vi "Scripting_SetConnectorPanePattern.vi"(0 "VIPath(s)/ViRef(s)":variant, 1 "Pattern":T1 items=["4x4x4", "5x6x5", "6x8x6"], 2 "UpdateCallersInThisClassOnly":string, 5 "error in (no error)":errorcluster, 6 "AppRef":refnum<vi>) -> (19 "error out":errorcluster)   [LabVIEW 2020]
uses:
  Scripting_ConnectorPanePatternType.ctl
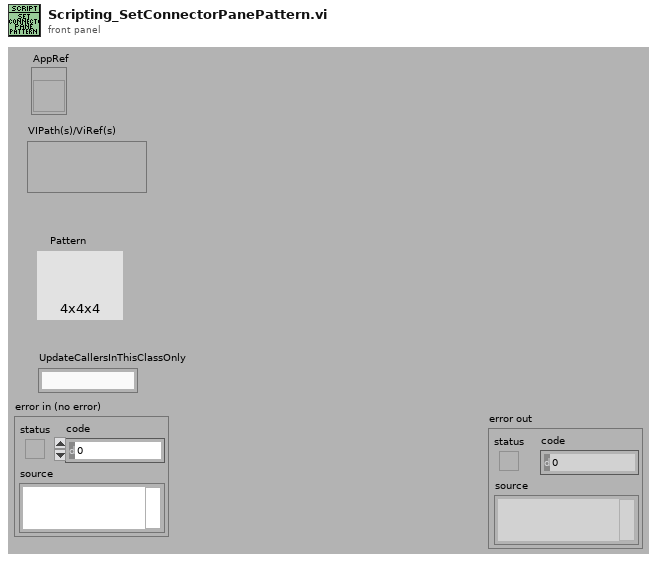
[diagram p1: front panel]
types:
  T1 = typedef "Scripting_ConnectorPanePatternType.ctl" = u16
  T2 = enum32{"invalid lock state", "Not Locked", "Locked (No Password)", "Password-protected"}
  T3 = enum32{"invalid VI type", "Standard VI", "Control VI", "Global VI", "Polymorphic VI", "Configuration VI", "SubSystem", "Facade VI", "Method VI", "Statechart Diagram VI"}
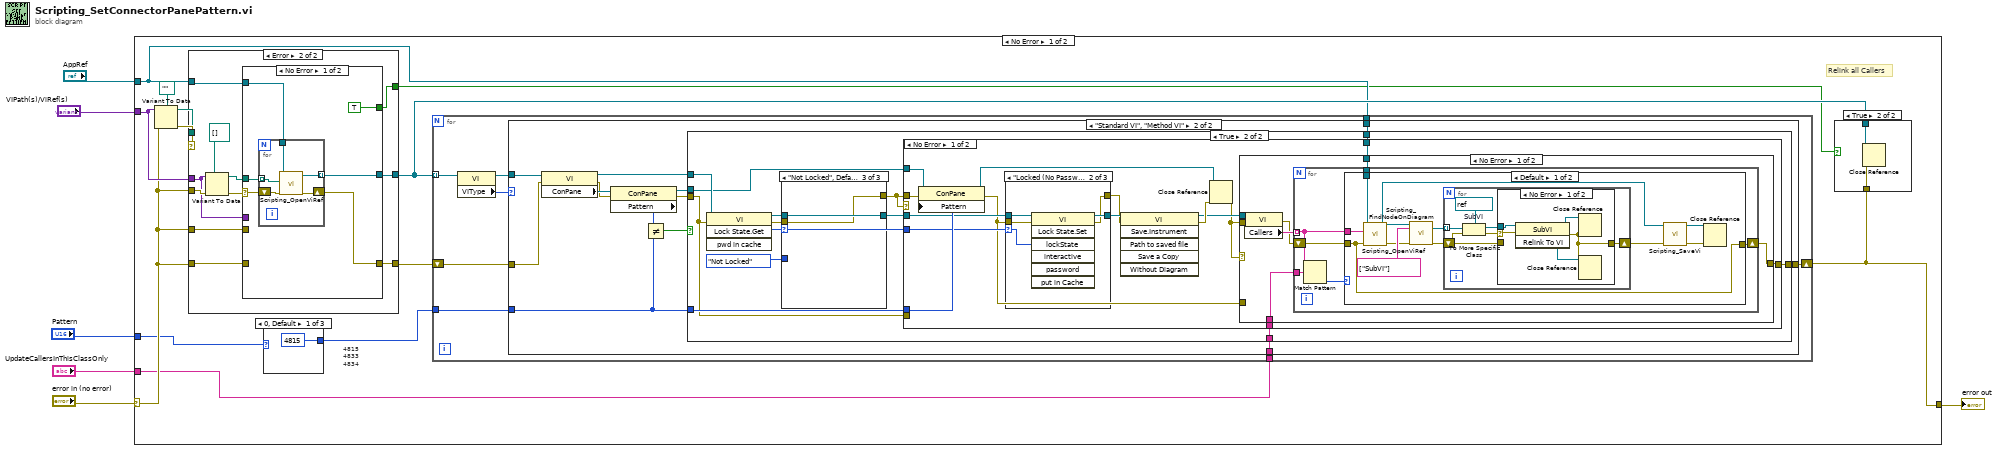
[diagram p0: block diagram]
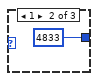
[diagram p3: hidden frame]
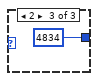
[diagram p4: hidden frame]
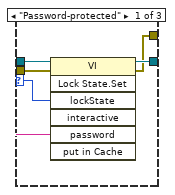
[diagram p10: hidden frame]
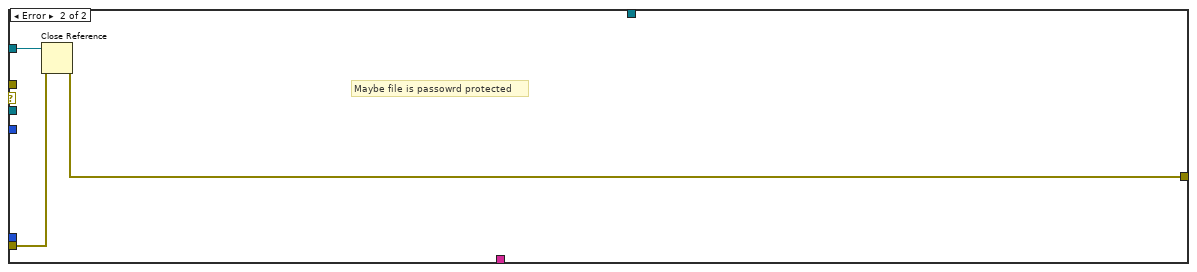
[diagram p12: hidden frame]
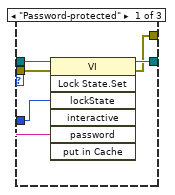
[diagram p13: hidden frame]
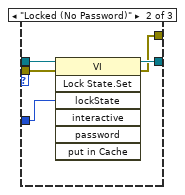
[diagram p14: hidden frame]
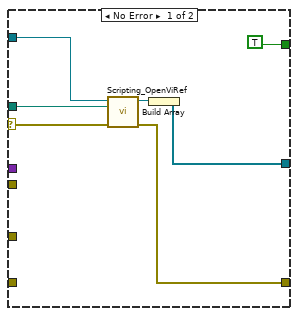
[diagram p15: hidden frame]
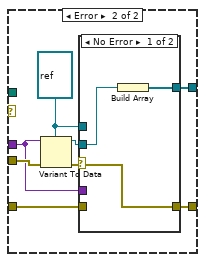
[diagram p16: hidden frame]
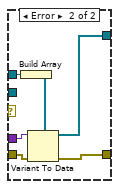
[diagram p17: hidden frame]
diagram:
  n1 = case shown="No Error" "error in (no error)" {
    selector: "error in (no error)" -> [w15 w189]
    tunnel: "VIPath(s)/ViRef(s)" -> [w17 _]
    tunnel: "Pattern" -> [w14 _]
    tunnel: [w8 w189] -> w3
    tunnel: "UpdateCallersInThisClassOnly" -> [w10 _]
    tunnel: "AppRef" -> [w9 _]
    frame No Error {
      # "Relink all Callers"
      # "4815\n4833\n4834"
      n2 = Variant To Data(error in=w15, type=path "", Variant=w17) -> (data=w16:path, error out=w18:errorcluster)
      n3 = case shown="Error" w18 {
        selector: w18 -> [w148 _]
        tunnel: w17 -> [_ w155]
        tunnel: w16 -> [w149 _]
        tunnel: [w146 w157] -> w11
        tunnel: w15 -> [_ w156]
        tunnel: w15 -> [_ w154]
        tunnel: w15 -> [_ w153]
        tunnel: [w145 w152] -> w12
        tunnel: [TRUE w151] -> w7
        tunnel: w9 -> [w143 w150]
        frame No Error {
          n4 = call "Scripting_OpenViRef.vi"("error in"=w148, "ViPath/ViName/Viref"=w149, "AppRef"=w143) -> ("error out"=w145:errorcluster, "vi reference"=w147:refnum<vi>)  [unwired: 6 in, 1 out]
          n5 = Build Array(w147) -> (w146:refnum<vi>[])
        }
        frame Error {
          n6 = Variant To Data(error in=w156, type=path[] [], Variant=w155) -> (data=w158:path[], error out=w159:errorcluster)
          n7 = case shown="No Error" w159 {
            selector: w159 -> [w164 _]
            tunnel: w158 -> [w166 _]
            tunnel: [w165 w177] -> w157
            tunnel: w155 -> [_ w174]
            tunnel: w154 -> [_ w179]
            tunnel: w153 -> [_ w175]
            tunnel: [w163 w172] -> w152
            tunnel: [TRUE _] -> w151
            tunnel: w150 -> [w161 _]
            frame No Error {
              n8 = for {
                tunnel: w166 -> [w171] mode=indexing
                tunnel: [w170] -> w165 mode=indexing
                shift-right: [w168] -> w163
                shift-left: w164 -> [w169]
                tunnel: w161 -> [w167]
                n9 = call "Scripting_OpenViRef.vi"("error in"=w169, "ViPath/ViName/Viref"=w171, "AppRef"=w167) -> ("error out"=w168:errorcluster, "vi reference"=w170:refnum<vi>)  [unwired: 6 in, 1 out]
              }
            }
            frame Error {
              w173 = refnum<vi> refnum ("Reference")
              n10 = Variant To Data(error in=w179, type=w173, Variant=w174) -> (data=w178:refnum<vi>, error out=w176:errorcluster)
              n11 = case shown="No Error" w176 {
                selector: w176 -> [w180 _]
                tunnel: w178 -> [w182 _]
                tunnel: [w181 w184] -> w177
                tunnel: w175 -> [_ w188]
                tunnel: w174 -> [_ w187]
                tunnel: w173 -> [_ w186]
                tunnel: [w180 w183] -> w172
                frame No Error {
                  n12 = Build Array(w182) -> (w181:refnum<vi>[])
                }
                frame Error {
                  n13 = Build Array(w186) -> (w185:refnum<vi>[])
                  n14 = Variant To Data(error in=w188, type=w185, Variant=w187) -> (data=w184:refnum<vi>[], error out=w183:errorcluster)
                }
              }
            }
          }
        }
      }
      n15 = case shown="0, Default" w14 {
        tunnel: [u32 4815 ("Pattern") u32 4833 ("Pattern") u32 4834 ("Pattern")] -> w13
        frame 0, Default {
        }
        frame 1 {
        }
        frame 2 {
        }
      }
      n16 = for {
        tunnel: w11 -> [w29] mode=indexing
        tunnel: w13 -> [w30]
        shift-right: [w31] -> w8
        shift-left: w12 -> [w32]
        tunnel: w10 -> [w26]
        tunnel: w9 -> [w25]
        n17 = property class="VI"(reference=w29) -> (reference out=w28:refnum<vi>, "VIType"=w27:T3)  [unwired: 1 in, 1 out]
        n18 = case shown="\"Standard VI\", \"Method VI\"" w27 {
          tunnel: w32 -> [w33 w42]
          tunnel: [w33 w39] -> w31
          tunnel: w30 -> [_ w38]
          tunnel: w28 -> [_ w37]
          tunnel: w26 -> [_ w35]
          tunnel: w25 -> [_ w34]
          frame "invalid VI type", "Control VI", "Polymorphic VI", Default {
          }
          frame "Standard VI", "Method VI" {
            n19 = property class="VI"(reference=w37, error in=w42) -> (reference out=w36:refnum<vi>, error out=w43:errorcluster, "ConPane"=w46:refnum<vi>)
            n20 = property class="ConPane"(reference=w46, error in=w43) -> (reference out=w45:refnum<vi>, error out=w44:errorcluster, "Pattern"=w41:u32)
            n21 = Not Equal?(x=w41, y=w38) -> (x != y?=w40:bool)
            n22 = case shown="True" w40 {
              tunnel: w45 -> [_ w55]
              tunnel: w44 -> [w47 w50]
              tunnel: [w47 w52] -> w39
              tunnel: w38 -> [_ w60]
              tunnel: w36 -> [_ w59]
              tunnel: w35 -> [_ w49]
              tunnel: w34 -> [_ w48]
              frame False {
              }
              frame True {
                n23 = invoke class="VI" method="Lock State.Get"(reference=w59, error in=w50) -> (reference out=w58:refnum<vi>, error out=w57:errorcluster, "Get Lock State"=w54:T2)  [unwired: 2 in, 1 out]
                n24 = case shown="\"Not Locked\", Default" w54 {
                  tunnel: w58 -> [w135 w140 w142]
                  tunnel: w57 -> [w134 w139 w141]
                  tunnel: T2."Not Locked" ("Lock State") -> [w133 w138 _]
                  tunnel: [w131 w137 w142] -> w53
                  tunnel: [w130 w136 w141] -> w51
                  frame "Password-protected" {
                    n25 = invoke class="VI" method="Lock State.Set"(reference=w135, error in=w134, "lockState"=w133, "password"="Endevo Knows Goop!" ("Password")) -> (reference out=w131:refnum<vi>, error out=w130:errorcluster)  [unwired: 3 in, 5 out]
                  }
                  frame "Locked (No Password)" {
                    (unwired) "Endevo Knows Goop!" ("Password")
                    n26 = invoke class="VI" method="Lock State.Set"(reference=w140, error in=w139, "lockState"=w138) -> (reference out=w137:refnum<vi>, error out=w136:errorcluster)  [unwired: 4 in, 5 out]
                  }
                  frame "Not Locked", Default {
                  }
                }
                n27 = case shown="No Error" w51 {
                  tunnel: w60 -> [w75 _]
                  tunnel: w51 -> [w74 _]
                  tunnel: w55 -> [w73 w129]
                  tunnel: w54 -> [w72 _]
                  tunnel: w53 -> [w67 _]
                  tunnel: [w65 w127] -> w52
                  tunnel: w50 -> [_ w128]
                  tunnel: w49 -> [w62 _]
                  tunnel: w48 -> [w61 _]
                  frame No Error {
                    n28 = property class="ConPane"(reference=w73, error in=w74, "Pattern"=w75) -> (reference out=w68:refnum<vi>, error out=w63:errorcluster)
                    n29 = case shown="\"Locked (No Password)\"" w72 {
                      selector: w72 -> [w114 w120 _]
                      tunnel: w67 -> [w119 w124 w126]
                      tunnel: w63 -> [w118 w123 w125]
                      tunnel: [w116 w122 w126] -> w71
                      tunnel: [w115 w121 w125] -> w70
                      frame "Password-protected" {
                        n30 = invoke class="VI" method="Lock State.Set"(reference=w119, error in=w118, "lockState"=w114, "password"="Endevo Knows Goop!" ("Password")) -> (reference out=w116:refnum<vi>, error out=w115:errorcluster)  [unwired: 3 in, 5 out]
                      }
                      frame "Locked (No Password)" {
                        (unwired) "Endevo Knows Goop!" ("Password")
                        n31 = invoke class="VI" method="Lock State.Set"(reference=w124, error in=w123, "lockState"=w120) -> (reference out=w122:refnum<vi>, error out=w121:errorcluster)  [unwired: 4 in, 5 out]
                      }
                      frame "Not Locked", Default {
                      }
                    }
                    n32 = invoke class="VI" method="Save.Instrument"(reference=w71, error in=w70) -> (reference out=w66:refnum<vi>, error out=w69:errorcluster)  [unwired: 4 in, 4 out]
                    n33 = Close Reference(reference=w68, error in (no error)=w69) -> (error out=w64:errorcluster)
                    n34 = case shown="No Error" w64 {
                      tunnel: w66 -> [w82 _]
                      tunnel: w64 -> [w81 _]
                      tunnel: [w78 w113] -> w65
                      tunnel: w63 -> [_ w113]
                      tunnel: w62 -> [w77 _]
                      tunnel: w61 -> [w76 _]
                      frame No Error {
                        n35 = property class="VI"(reference=w82, error in=w81) -> (error out=w79:errorcluster, "Callers"=w80:string[])  [unwired: 1 out]
                        n36 = for {
                          tunnel: w80 -> [w86] mode=indexing
                          shift-right: [w87] -> w78
                          shift-left: w79 -> [w88]
                          tunnel: w77 -> [w85]
                          tunnel: w76 -> [w83]
                          n37 = Match Pattern(string=w86, regular expression=w85) -> (offset past match=w84:i32)  [unwired: 1 in, 3 out]
                          n38 = case shown="Default" w84 {
                            tunnel: w88 -> [w90 w112]
                            tunnel: [w90 w112] -> w87
                            tunnel: w86 -> [w91 _]
                            tunnel: w83 -> [w89 _]
                            frame Default {
                              n39 = call "Scripting_OpenViRef.vi"("error in"=w90, "ViPath/ViName/Viref"=w91, "AppRef"=w89) -> ("error out"=w98:errorcluster, "vi reference"=w93:refnum<vi>)  [unwired: 6 in, 1 out]
                              n40 = call "Scripting_FindNodeOnDiagram.vi"("ViRef(Ignored If Not Wired)"=w93, "NodeTypesToSearchFor"=string[] ["SubVI"], "error in (no error)"=w98) -> ("Nodes"=w96:refnum<vi>[], "error out"=w97:errorcluster)  [unwired: 15 in]
                              n41 = for {
                                shift-right: [w102] -> w95
                                shift-left: w97 -> [w100]
                                tunnel: w96 -> [w105] mode=indexing
                                w104 = refnum<vi> refnum  # SubVI
                                n42 = To More Specific Class(target class=w104, reference=w105, error in=w100) -> (specific class reference=w103:refnum<vi>, error out=w101:errorcluster)
                                n43 = case shown="No Error" w101 {
                                selector: w101 -> [w106 _]
                                tunnel: w103 -> [w110 _]
                                tunnel: [w107 w111] -> w102
                                tunnel: w100 -> [_ w111]
                                frame No Error {
                                n44 = invoke class="SubVI" method="Relink To VI"(reference=w110, error in=w106) -> (reference out=w108:refnum<vi>, error out=w107:errorcluster, "Relink To VI"=w109:refnum<vi>)  [unwired: 1 in]
                                n45 = Close Reference(reference=w108, error in (no error)=w107) -> ()  [unwired: 1 out]
                                n46 = Close Reference(reference=w109, error in (no error)=w107) -> ()  [unwired: 1 out]
                                }
                                frame Error {
                                }
                                }
                              }
                              n47 = call "Scripting_SaveVi.vi"("error in (no error)"=w95, "VIRefToSaveIn"=w93) -> ("error out"=w94:errorcluster, "VIRefToSaveOut"=w92:refnum<vi>)  [unwired: 8 in]
                              n48 = Close Reference(reference=w92, error in (no error)=w94) -> ()  [unwired: 1 out]
                            }
                            frame -1 {
                            }
                          }
                        }
                      }
                      frame Error {
                        # "Maybe file is read only"
                      }
                    }
                  }
                  frame Error {
                    # "Maybe file is passowrd protected"
                    n49 = Close Reference(reference=w129, error in (no error)=w128) -> (error out=w127:errorcluster)
                  }
                }
              }
            }
          }
        }
      }
      n50 = case shown="True" w7 {
        tunnel: w11 -> [_ w21]
        tunnel: w8 -> [_ w20]
        frame False {
        }
        frame True {
          n51 = Close Reference(reference=w21, error in (no error)=w20) -> ()  [unwired: 1 out]
        }
      }
    }
    frame Error {
    }
  }
  "error out" <- w3
